vi "夹爪压力保存.vi"(8 "error in (no error)":errorcluster caption="错误输入（无错误）", 9 "DB5000.R":T1, 10 "DB5000.X":T2, 11 "夹爪数组in":dbl[][](array[numeric])) -> (0 "字符串":string, 1 "夹爪10压力值":sgl, 2 "夹爪压力值":dbl[](array[numeric]), 3 "夹爪数组out":dbl[][](array[numeric]), 4 "error out":errorcluster caption="错误输出")   [LabVIEW 2017]
panel:
  out "添加的数组 19":dbl[](array[numeric])
  out "夹爪2":dbl format="%#_3g"
  out "添加的数组 20":dbl[](array[numeric])
  out "夹爪1":dbl format="%#_3g"
  out "添加的数组 17":dbl[](array[numeric])
  out "夹爪3":dbl format="%#_3g"
  out "添加的数组 8":dbl[](array[numeric])
  out "夹爪10":dbl format="%#_3g"
  out "添加的数组 7":dbl[](array[numeric])
  out "夹爪9":dbl format="%#_3g"
  out "添加的数组 6":dbl[](array[numeric])
  out "夹爪8":dbl format="%#_3g"
  out "添加的数组 5":dbl[](array[numeric])
  out "夹爪7":dbl format="%#_3g"
  out "添加的数组 4":dbl[](array[numeric])
  out "夹爪6":dbl format="%#_3g"
  out "添加的数组 3":dbl[](array[numeric])
  out "夹爪5":dbl format="%#_3g"
  out "添加的数组 2":dbl[](array[numeric])
  out "夹爪4":dbl format="%#_3g"
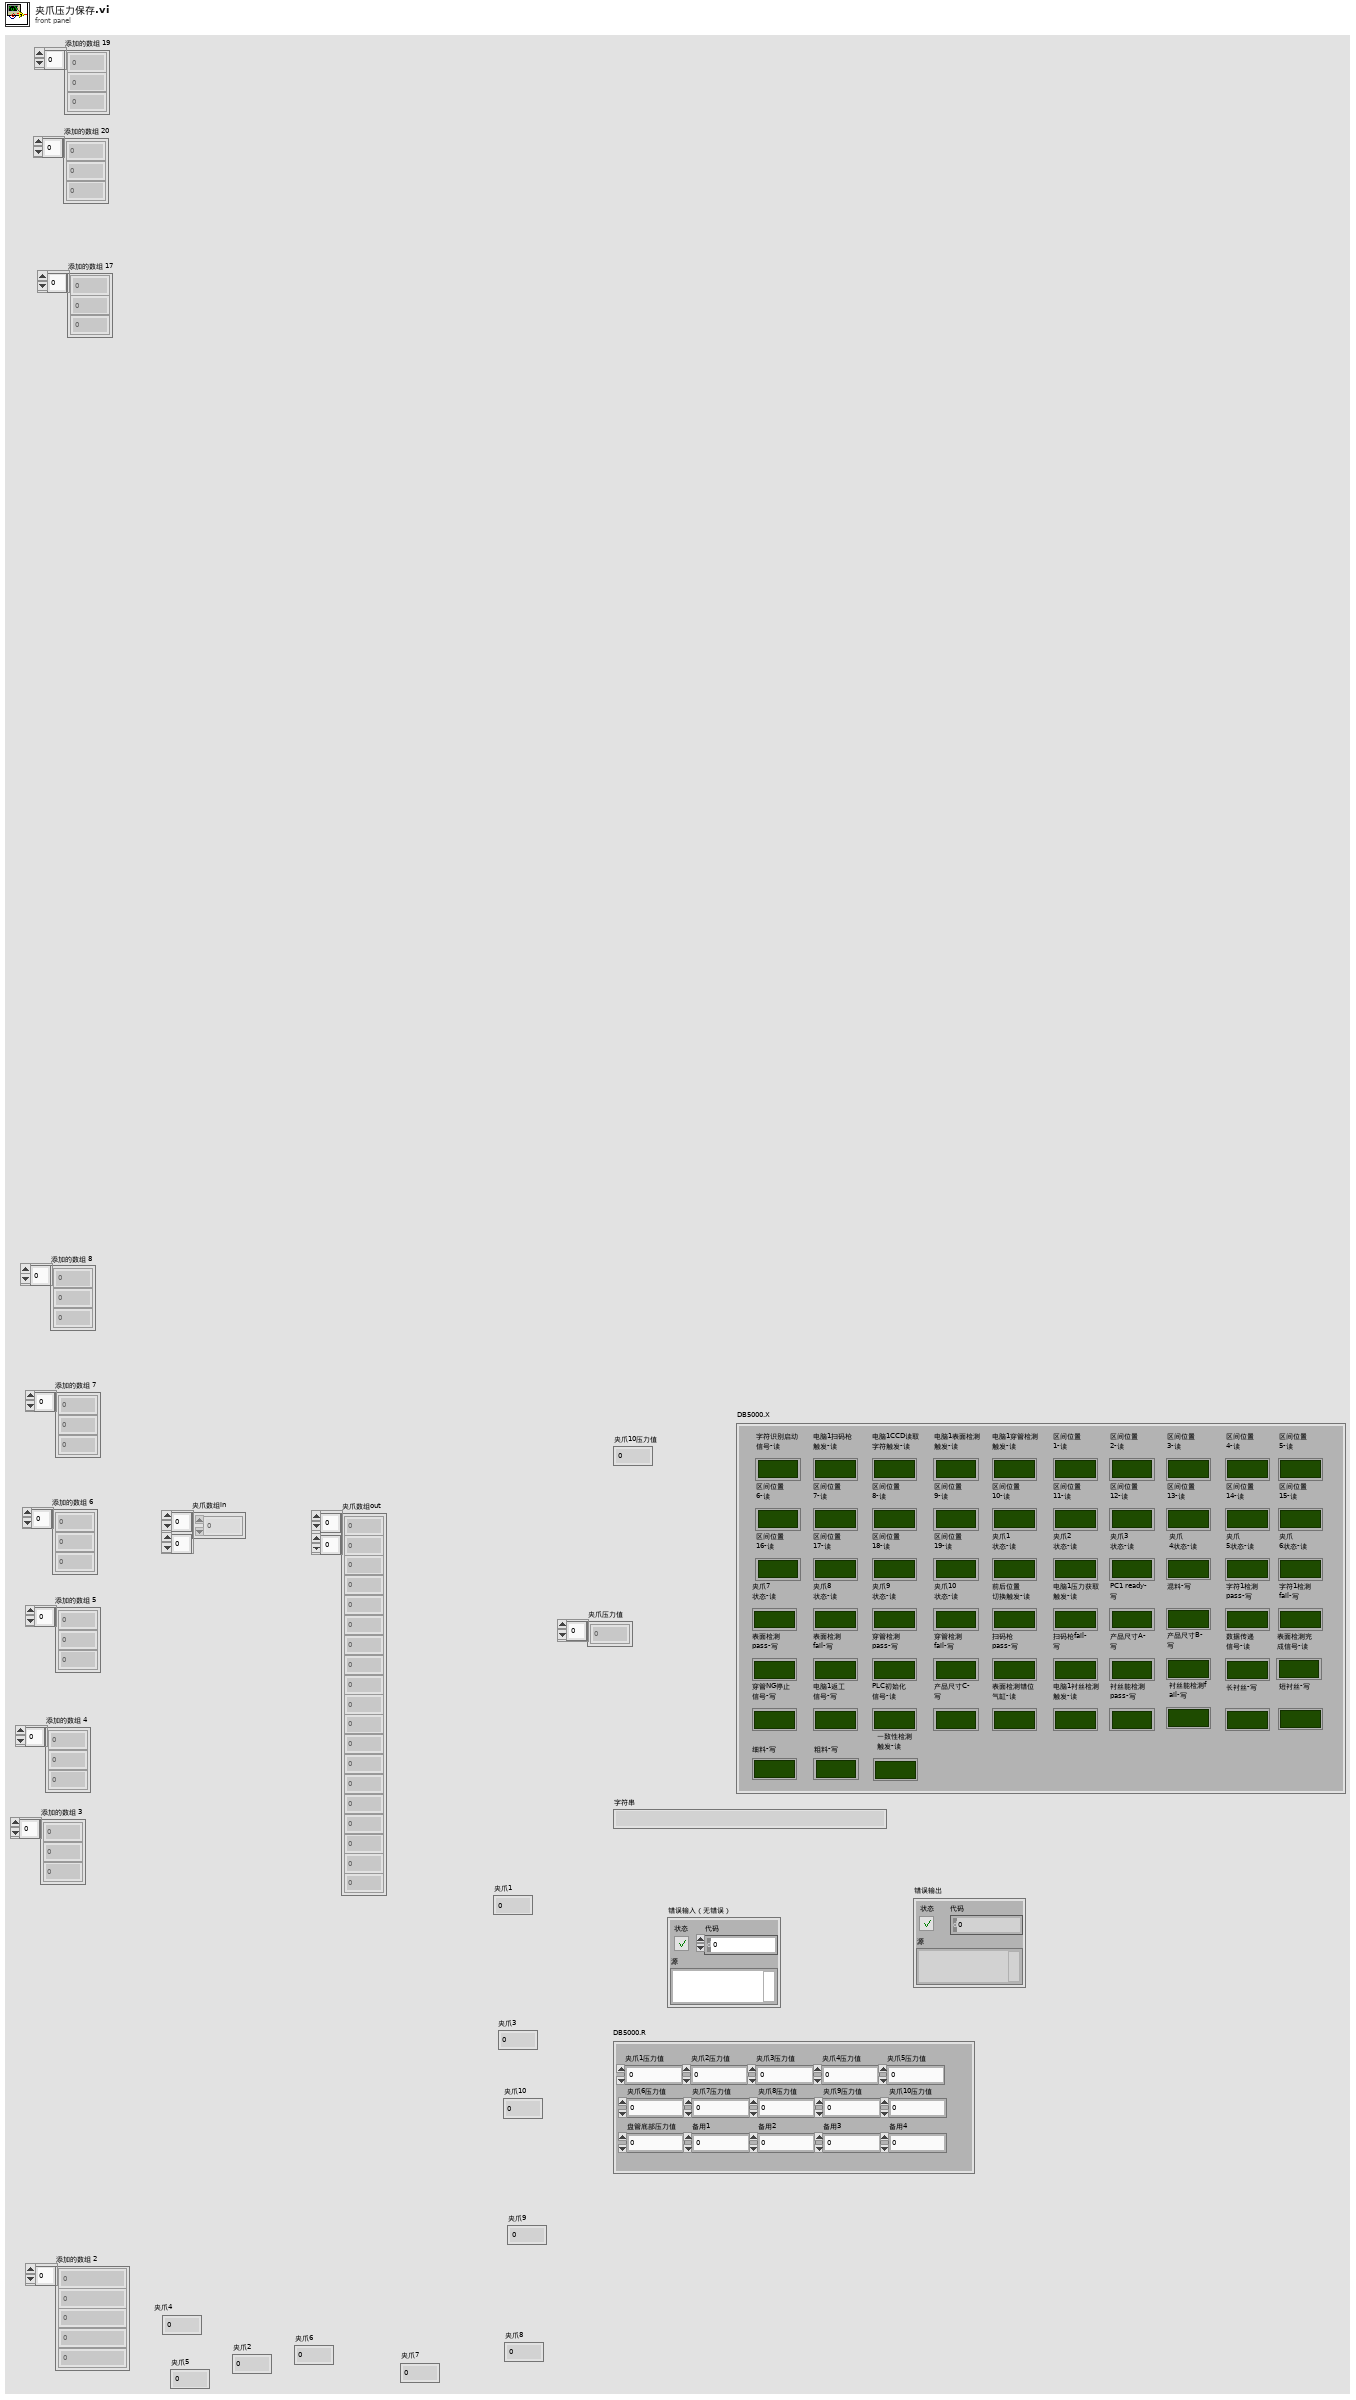
[diagram p1: front panel]
types:
  T1 = cluster{"夹爪1压力值":sgl, "夹爪2压力值":sgl, "夹爪3压力值":sgl, "夹爪4压力值":sgl, "夹爪5压力值":sgl, "夹爪6压力值":sgl, "夹爪7压力值":sgl, "夹爪8压力值":sgl, "夹爪9压力值":sgl, "夹爪10压力值":sgl, "盘管底部压力值":sgl, "备用1":sgl, "备用2":sgl, "备用3":sgl, "备用4":sgl}
  T2 = cluster{"字符识别启动\n信号-读":bool, "电脑1扫码枪\n触发-读":bool, "电脑1CCD读取\n字符触发-读":bool, "电脑1表面检测\n触发-读":bool, "电脑1穿管检测\n触发-读":bool, "区间位置\n1-读":bool, "区间位置\n2-读":bool, "区间位置\n3-读":bool, "区间位置\n4-读":bool, "区间位置\n5-读":bool, "区间位置\n6-读":bool, "区间位置\n7-读":bool, "区间位置\n8-读":bool, "区间位置\n9-读":bool, "区间位置\n10-读":bool, "区间位置\n11-读":bool, "区间位置\n12-读":bool, "区间位置\n13-读":bool, "区间位置\n14-读":bool, "区间位置\n15-读":bool, "区间位置\n16-读":bool, "区间位置\n17-读":bool, "区间位置\n18-读":bool, "区间位置\n19-读":bool, "夹爪1\n状态-读":bool, "夹爪2\n状态-读":bool, "夹爪3\n状态-读":bool, "夹爪\n4状态-读":bool, "夹爪\n5状态-读":bool, "夹爪\n6状态-读":bool, "夹爪7\n状态-读":bool, "夹爪8\n状态-读":bool, "夹爪9\n状态-读":bool, "夹爪10\n状态-读":bool, "前后位置\n切换触发-读":bool, "电脑1压力获取\n触发-读":bool, "PC1 ready-\n写 ":bool, "混料-写\n":bool, "字符1检测\npass-写":bool, "字符1检测\nfail-写":bool, "表面检测\npass-写":bool, "表面检测\nfail-写":bool, "穿管检测\npass-写":bool, "穿管检测\nfail-写":bool, "扫码枪\npass-写":bool, "扫码枪fail-\n写":bool, "产品尺寸A-\n写":bool, "产品尺寸B-\n写":bool, "数据传递\n信号-读":bool, "表面检测完\n成信号-读":bool, "穿管NG停止\n信号-写":bool, "电脑1返工\n信号-写":bool, "PLC初始化\n信号-读":bool, "产品尺寸C-\n写":bool, "表面检测错位\n气缸-读":bool, "电脑1衬丝检测\n触发-读":bool, "衬丝能检测\npass-写":bool, "衬丝能检测f\nail-写":bool, "长衬丝-写\n":bool, "短衬丝-写\n":bool, "细料-写":bool, "粗料-写":bool, "一致性检测\n触发-读":bool}
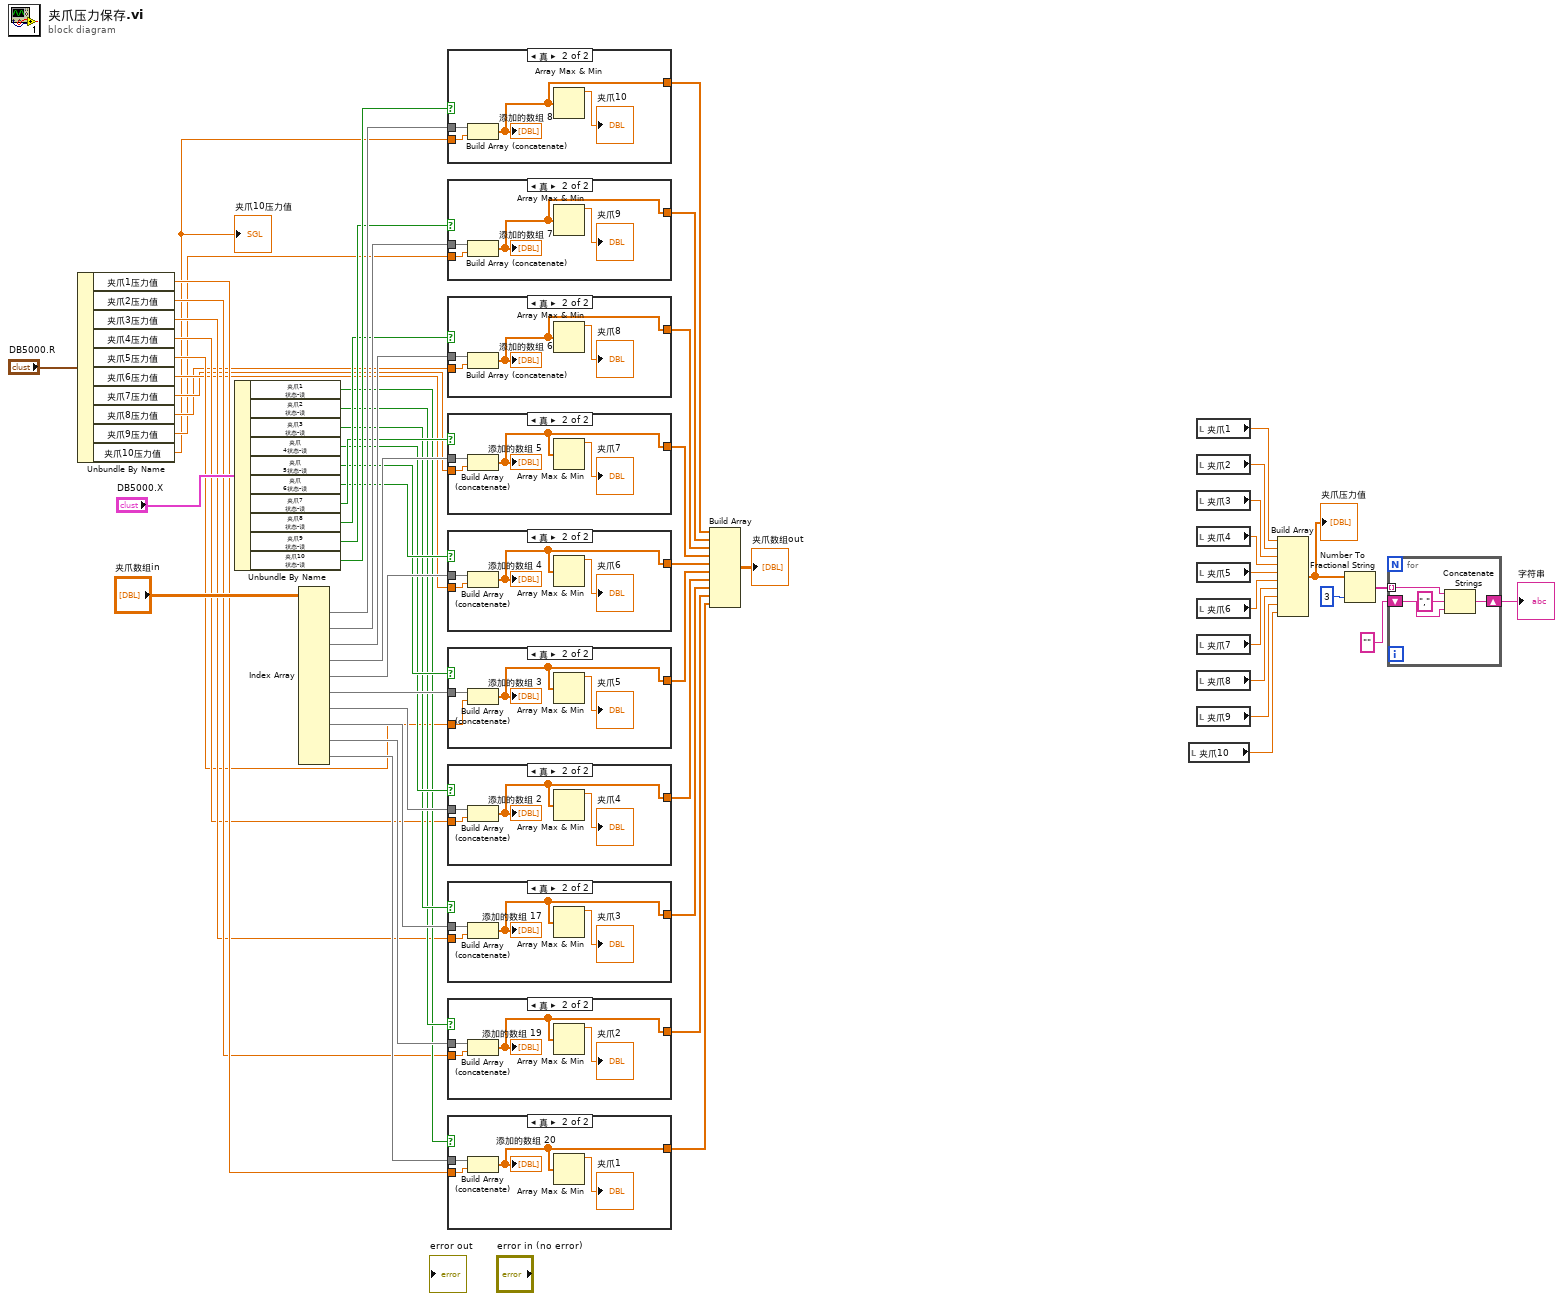
[diagram p0: block diagram]
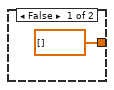
[diagram p2: hidden frame]
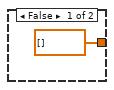
[diagram p3: hidden frame]
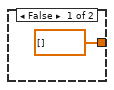
[diagram p4: hidden frame]
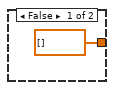
[diagram p5: hidden frame]
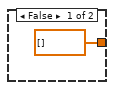
[diagram p6: hidden frame]
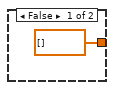
[diagram p7: hidden frame]
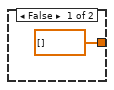
[diagram p8: hidden frame]
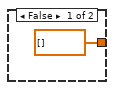
[diagram p9: hidden frame]
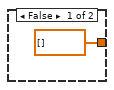
[diagram p10: hidden frame]
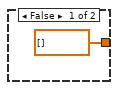
[diagram p11: hidden frame]
diagram:
  n1 = Unbundle By Name("DB5000.R") -> ("夹爪1压力值"=w10:sgl, "夹爪2压力值"=w9:sgl, "夹爪3压力值"=w8:sgl, "夹爪4压力值"=w7:sgl, "夹爪5压力值"=w6:sgl, "夹爪6压力值"=w5:sgl, "夹爪7压力值"=w4:sgl, "夹爪8压力值"=w3:sgl, "夹爪9压力值"=w2:sgl, "夹爪10压力值"=w1:sgl)
  "夹爪10压力值" <- w1
  n2 = Unbundle By Name("DB5000.X") -> ("夹爪1\n状态-读"=w12:bool, "夹爪2\n状态-读"=w13:bool, "夹爪3\n状态-读"=w14:bool, "夹爪\n4状态-读"=w15:bool, "夹爪\n5状态-读"=w16:bool, "夹爪\n6状态-读"=w17:bool, "夹爪7\n状态-读"=w18:bool, "夹爪8\n状态-读"=w19:bool, "夹爪9\n状态-读"=w20:bool, "夹爪10\n状态-读"=w21:bool)
  n3 = Index Array(array="夹爪数组in") -> (element #1=w48:dbl[], element #2=w47:dbl[], element #3=w46:dbl[], element #4=w45:dbl[], element #5=w44:dbl[], element #6=w43:dbl[], element #7=w42:dbl[], element #8=w41:dbl[], element #9=w40:dbl[], element #10=w39:dbl[])  [unwired: 20 in]
  n4 = case shown="真" w21 {
    tunnel: [dbl[] [] ("添加的数组") w62] -> w38
    tunnel: w1 -> [_ w64]
    tunnel: w48 -> [_ w61]
    frame False {
    }
    frame True {
      n5 = Build Array (concatenate)(w61, w64) -> (w62:dbl[])
      "添加的数组 8" <- w62
      n6 = Array Max & Min(array=w62) -> (max value=→"夹爪10":dbl)  [unwired: 3 out]
    }
  }
  n7 = case shown="真" w20 {
    tunnel: [dbl[] [] ("添加的数组") w67] -> w37
    tunnel: w2 -> [_ w69]
    tunnel: w47 -> [_ w66]
    frame False {
    }
    frame True {
      n8 = Build Array (concatenate)(w66, w69) -> (w67:dbl[])
      "添加的数组 7" <- w67
      n9 = Array Max & Min(array=w67) -> (max value=→"夹爪9":dbl)  [unwired: 3 out]
    }
  }
  n10 = case shown="真" w19 {
    tunnel: [dbl[] [] ("添加的数组") w72] -> w36
    tunnel: w3 -> [_ w74]
    tunnel: w46 -> [_ w71]
    frame False {
    }
    frame True {
      n11 = Build Array (concatenate)(w71, w74) -> (w72:dbl[])
      "添加的数组 6" <- w72
      n12 = Array Max & Min(array=w72) -> (max value=→"夹爪8":dbl)  [unwired: 3 out]
    }
  }
  n13 = case shown="真" w18 {
    tunnel: [dbl[] [] ("添加的数组") w77] -> w35
    tunnel: w4 -> [_ w79]
    tunnel: w45 -> [_ w76]
    frame False {
    }
    frame True {
      n14 = Build Array (concatenate)(w76, w79) -> (w77:dbl[])
      "添加的数组 5" <- w77
      n15 = Array Max & Min(array=w77) -> (max value=→"夹爪7":dbl)  [unwired: 3 out]
    }
  }
  n16 = case shown="真" w17 {
    tunnel: [dbl[] [] ("添加的数组") w82] -> w34
    tunnel: w5 -> [_ w84]
    tunnel: w44 -> [_ w81]
    frame False {
    }
    frame True {
      n17 = Build Array (concatenate)(w81, w84) -> (w82:dbl[])
      "添加的数组 4" <- w82
      n18 = Array Max & Min(array=w82) -> (max value=→"夹爪6":dbl)  [unwired: 3 out]
    }
  }
  n19 = case shown="真" w16 {
    tunnel: [dbl[] [] ("添加的数组") w87] -> w33
    tunnel: w6 -> [_ w89]
    tunnel: w43 -> [_ w86]
    frame False {
    }
    frame True {
      n20 = Build Array (concatenate)(w86, w89) -> (w87:dbl[])
      "添加的数组 3" <- w87
      n21 = Array Max & Min(array=w87) -> (max value=→"夹爪5":dbl)  [unwired: 3 out]
    }
  }
  n22 = case shown="真" w15 {
    tunnel: [dbl[] [] ("添加的数组") w93] -> w32
    tunnel: w7 -> [_ w94]
    tunnel: w42 -> [_ w91]
    frame False {
    }
    frame True {
      n23 = Build Array (concatenate)(w91, w94) -> (w93:dbl[])
      "添加的数组 2" <- w93
      n24 = Array Max & Min(array=w93) -> (max value=→"夹爪4":dbl)  [unwired: 3 out]
    }
  }
  n25 = case shown="真" w14 {
    tunnel: [dbl[] [] ("添加的数组") w97] -> w31
    tunnel: w8 -> [_ w99]
    tunnel: w41 -> [_ w96]
    frame False {
    }
    frame True {
      n26 = Build Array (concatenate)(w96, w99) -> (w97:dbl[])
      "添加的数组 17" <- w97
      n27 = Array Max & Min(array=w97) -> (max value=→"夹爪3":dbl)  [unwired: 3 out]
    }
  }
  n28 = case shown="真" w13 {
    tunnel: [dbl[] [] ("添加的数组") w102] -> w30
    tunnel: w9 -> [_ w104]
    tunnel: w40 -> [_ w101]
    frame False {
    }
    frame True {
      n29 = Build Array (concatenate)(w101, w104) -> (w102:dbl[])
      "添加的数组 19" <- w102
      n30 = Array Max & Min(array=w102) -> (max value=→"夹爪2":dbl)  [unwired: 3 out]
    }
  }
  n31 = case shown="真" w12 {
    tunnel: [dbl[] [] ("添加的数组") w108] -> w29
    tunnel: w10 -> [_ w109]
    tunnel: w39 -> [_ w106]
    frame False {
    }
    frame True {
      n32 = Build Array (concatenate)(w106, w109) -> (w108:dbl[])
      "添加的数组 20" <- w108
      n33 = Array Max & Min(array=w108) -> (max value=→"夹爪1":dbl)  [unwired: 3 out]
    }
  }
  n34 = Build Array(w38, w37, w36, w35, w34, w33, w32, w31, w30, w29) -> (→"夹爪数组out":dbl[][])
  n35 = local read "夹爪10"() -> (w50:dbl)
  n36 = local read "夹爪1"() -> (w59:dbl)
  n37 = local read "夹爪2"() -> (w58:dbl)
  n38 = local read "夹爪3"() -> (w57:dbl)
  n39 = local read "夹爪4"() -> (w56:dbl)
  n40 = local read "夹爪5"() -> (w55:dbl)
  n41 = local read "夹爪6"() -> (w54:dbl)
  n42 = local read "夹爪7"() -> (w53:dbl)
  n43 = local read "夹爪8"() -> (w52:dbl)
  n44 = local read "夹爪9"() -> (w51:dbl)
  n45 = Build Array(w59, w58, w57, w56, w55, w54, w53, w52, w51, w50) -> (w27:dbl[])
  "夹爪压力值" <- w27
  n46 = Number To Fractional String(number=w27, precision (6)=i16 3 ("精度(6)")) -> (F-format string=w25:string[])  [unwired: 2 in]
  n47 = for {
    tunnel: w25 -> [w113] mode=indexing
    shift-right: [w110] -> w23
    shift-left: "" ("字符串") -> [w111]
    n48 = Concatenate Strings(w113, "," ("字符串"), w111) -> (w110:string)
  }
  "字符串" <- w23
